vi "Convert dB to Linear Ratio.vi"(4 "dB":dbl format="%.2f") -> (1 "X":dbl format="%.2f")   [LabVIEW 2011]
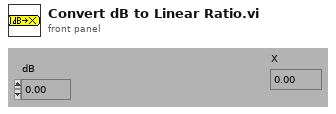
[diagram p1: front panel]
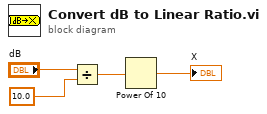
[diagram p0: block diagram]
diagram:
  n1 = Divide(x="dB", y=10.0) -> (x/y=w3:dbl)
  n2 = Power Of 10(x=w3) -> (10^x=→"X":dbl)
